vi "Leaktest Temp PID Control 02.vi"(4 "Control Mode":cluster{"Pos'n 1":T2, "Pos'n 2":T2}, 5 "process variable":dbl[](array[numeric])=[0.0] format="%.2f", 6 "dt (s)":dbl=-1.0 format="%.3f", 7 "Manual %":cluster{"Man 1":dbl, "Man 2":dbl} {"Man 2" format="%.1f"; "Man 1" format="%.1f"}, 8 "output range":cluster{"output high":dbl, "output low":dbl}={"output high"=100.0, "output low"=0.0}, 9 "Control Params":T1={"Warm Setpt C"=25.0, "WarmPID"={" gain (Kc)"=-10.0, "integral min"=0.5, "derivative min"=0.0}} {"Warm Setpt C" format="%.2f"; "WarmPID"."derivative min" format="%.3f"; "WarmPID"."integral min" format="%.3f"; "WarmPID"."gain (Kc)" format="%.3f"}) -> (3 "Output %":dbl[](array[numeric]))   [LabVIEW 2020]
uses:
  Leaktest Temp Mode Select Enum.ctl
  NI_PID_pid.lvlib
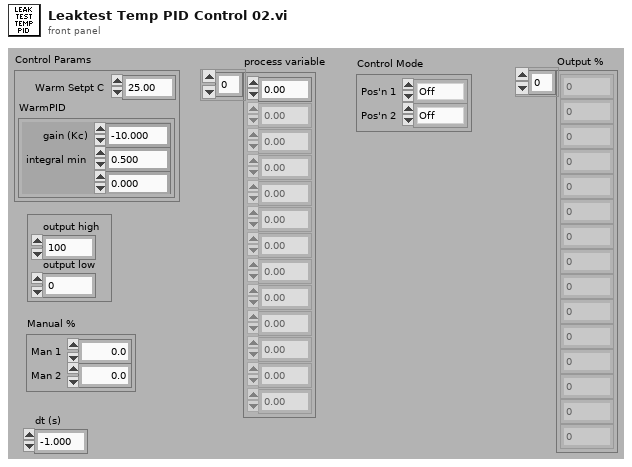
[diagram p1: front panel]
types:
  T1 = cluster{"Warm Setpt C":dbl, "WarmPID":cluster{" gain (Kc)":dbl, "integral min":dbl, "derivative min":dbl}}
  T2 = typedef "Leaktest Temp Mode Select Enum.ctl" = enum16{"Off", "Manual", "Auto"}
  T3 = cluster{" gain (Kc)":dbl, "integral min":dbl, "derivative min":dbl}
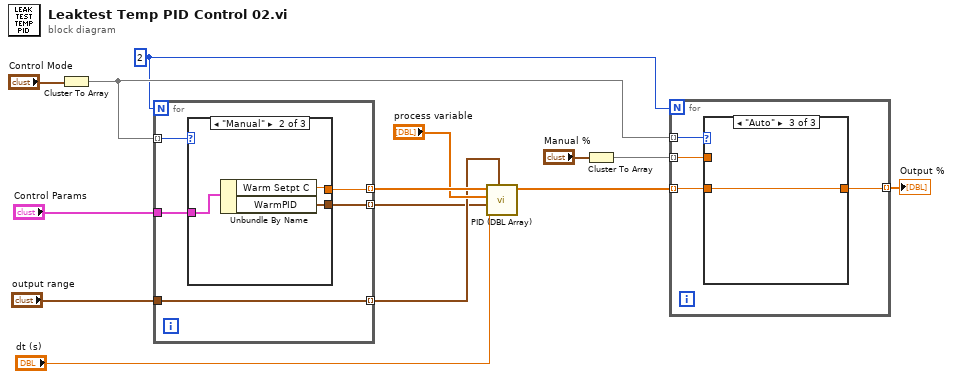
[diagram p0: block diagram]
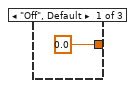
[diagram p2: hidden frame]
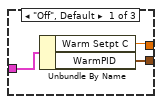
[diagram p4: hidden frame]
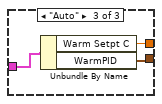
[diagram p5: hidden frame]
diagram:
  w3 = 2
  n1 = Cluster To Array(cluster="Control Mode") -> (array=w10:T2[])
  n2 = for {
    N: w3 -> [_]
    tunnel: w10 -> [w16] mode=indexing
    tunnel: [w19] -> w2 mode=indexing
    tunnel: "Control Params" -> [w18]
    tunnel: [w17] -> w12 mode=indexing
    tunnel: [w15] -> w4 mode=indexing
    tunnel: "output range" -> [w15]
    n3 = case shown="\"Manual\"" w16 {
      tunnel: [w21 w23 w26] -> w19
      tunnel: w18 -> [w22 w25 w28]
      tunnel: [w20 w24 w27] -> w17
      frame "Off", Default {
        n4 = Unbundle By Name(w22) -> ("Warm Setpt C"=w20:dbl, "WarmPID"=w21:T3)
      }
      frame "Manual" {
        n5 = Unbundle By Name(w25) -> ("Warm Setpt C"=w24:dbl, "WarmPID"=w23:T3)
      }
      frame "Auto" {
        n6 = Unbundle By Name(w28) -> ("Warm Setpt C"=w27:dbl, "WarmPID"=w26:T3)
      }
    }
  }
  n7 = call "PID (DBL Array).vi"("output range"=w4, "dt (s)"="dt (s)", "PID gains"=w2, "process variable"="process variable", "setpoint"=w12) -> ("output"=w9:dbl[])  [unwired: 5 in, 1 out]
  n8 = Cluster To Array(cluster="Manual %") -> (array=w7:dbl[])
  n9 = for {
    N: w3 -> [_]
    tunnel: w10 -> [w32] mode=indexing
    tunnel: [w31] -> w6 mode=indexing
    tunnel: w9 -> [w30] mode=indexing
    tunnel: w7 -> [w29] mode=indexing
    n10 = case shown="\"Auto\"" w32 {
      tunnel: [0.0 ("output") w34 w35] -> w31
      tunnel: w30 -> [_ _ w35]
      tunnel: w29 -> [_ w34 _]
      frame "Off", Default {
      }
      frame "Manual" {
      }
      frame "Auto" {
      }
    }
  }
  "Output %" <- w6
